vi "Lambda Percentage Flow (Read).vi"(6 "ISOBUS address":T1=-1 caption="ISOBUS address (-1)", 8 "error in":errorcluster, 11 "Mercury Reference In":T4) -> (0 "error out":errorcluster, 1 "Unit":T2, 2 "Target Open":dbl min=0.0 max=100.0 format="%#.1g", 3 "Mercury Reference Out":T4, 4 "Valid?":T3)   [LabVIEW 2016, in "Mercury iXX.lvlib" / "Lambda.lvlib"]
doc: "Check the percentage of the flow output associated with control loop."
uses:
  Lambda.lvlib
  Controls/Mercury Reference.ctl
  Controls/Comms Transport Layer.ctl
  Private/Controls/Query Dynamic Reference.ctl
  Controls/Is Valid LED.ctl
  Controls/Unit String.ctl
  Controls/ISOBus Address.ctl
  Private/Controls/Command Verbs.ctl
  Mercury iXX.lvlib
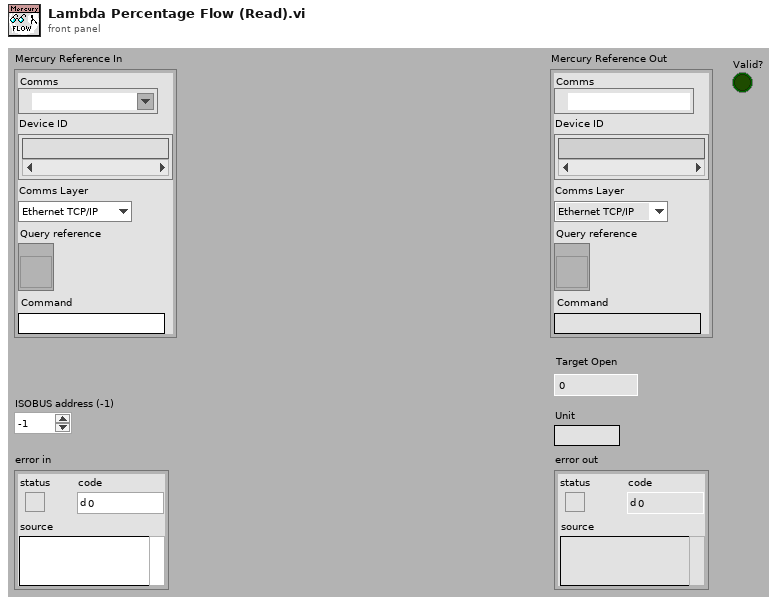
[diagram p1: front panel]
types:
  T1 = typedef "Mercury iXX.lvlib/ISOBus Address.ctl" = i32
  T2 = typedef "Mercury iXX.lvlib/Unit String.ctl" = string
  T3 = typedef "Mercury iXX.lvlib/Is Valid LED.ctl" = bool
  T4 = typedef "Mercury iXX.lvlib/Mercury Reference.ctl" = cluster{"Comms":refnum<visa-resource-name>, "Device ID":string[], "Comms Layer":T5, "Command":string, "Query reference":T6}
  T5 = typedef "Mercury iXX.lvlib/Comms Transport Layer.ctl" = enum16{"Ethernet TCP/IP", "USB", "ISOBus - RS-232", "GPIB"}
  T6 = typedef "Mercury iXX.lvlib/Query Dynamic Reference.ctl" = refnum<vi>
  T7 = typedef "Mercury iXX.lvlib/Command Verbs.ctl" = string
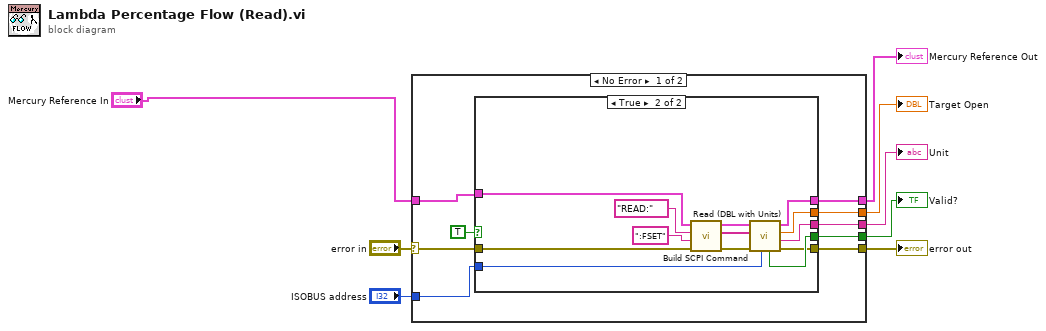
[diagram p0: block diagram]
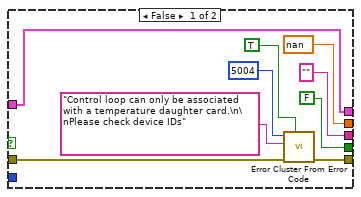
[diagram p2: hidden frame]
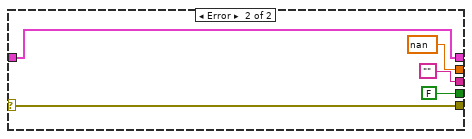
[diagram p3: hidden frame]
diagram:
  n1 = case shown="No Error" "error in" {
    selector: "error in" -> [w9 w44]
    tunnel: [w17 w40] -> w2
    tunnel: [w15 w44] -> w6
    tunnel: "ISOBUS address" -> [w16 _]
    tunnel: [w12 nan ("Scaled Value")] -> w3
    tunnel: [w14 FALSE ("Valid?")] -> w5
    tunnel: [w13 ""] -> w4
    tunnel: "Mercury Reference In" -> [w10 w40]
    frame No Error {
      n2 = case shown="True" TRUE {
        tunnel: w10 -> [w26 w33]
        tunnel: [w26 w28] -> w17
        tunnel: w9 -> [w24 w34]
        tunnel: w16 -> [_ w32]
        tunnel: [w25 w27] -> w15
        tunnel: [T3 FALSE ("Valid?") w31] -> w14
        tunnel: [T2 "" ("Unit") w30] -> w13
        tunnel: [nan ("Data (Dbl)") w29] -> w12
        frame False {
          n3 = call <vilib>:"Error Cluster From Error Code.vi"("show call chain? (False)"=TRUE, "error in (no error)"=w24, "error message (\"\")"="Control loop can only be associated with a temperature daughter card.\n\nPlease check device IDs" ("error message (\"\")"), "error code (0)"=5004) -> ("error out"=w25:errorcluster)  [unwired: 5 out]
        }
        frame True {
          n4 = call "Build SCPI Command.vi"("error in"=w34, "Noun(s)"=":FSET" ("Command"), "Verb"=T7 "READ:", "Mercury Reference In"=w33) -> ("error out"=w35:errorcluster, "SCPI Message(s)"=w37:string[], "Mercury Reference Out"=w38:T4)  [unwired: 5 out]
          n5 = call "Read (DBL with Units).vi"("ISOBUS address"=w32, "error in"=w35, "SCPI Message(s)"=w37, "Mercury Reference In"=w38) -> ("error out"=w27:errorcluster, "Unit"=w30:T2, "Data (Dbl)"=w29:dbl, "Mercury Reference Out"=w28:T4, "Valid?"=w31:T3)  [unwired: 3 out]
        }
      }
    }
    frame Error {
    }
  }
  "Mercury Reference Out" <- w2
  "Target Open" <- w3
  "Valid?" <- w5
  "Unit" <- w4
  "error out" <- w6
